vi "Inject Attribute List.vi"(6 "Attributes Ref":refnum<data-value>, 8 "error in (no error)":errorcluster, 11 "Start High Pressure Wash in":refnum<class "Start High Pressure Wash.lvclass">) -> (0 "error out":errorcluster, 3 "Start High Pressure Wash out":refnum<class "Start High Pressure Wash.lvclass">)   [LabVIEW 2019, in "Start High Pressure Wash.lvclass"]
uses:
  <vilib>/gpm_packages/@cs/Car-wash/Source/Process Steps/Start High Pressure Wash/Start High Pressure Wash.lvclass
  <vilib>/gpm_packages/@cs/lookup-table/Source/LookupTable/LookupTable.lvclass
  <vilib>/gpm_packages/@cs/lookup-table/Source/LookupTable/LookupTable.lvclass/LookupTable.ctl
  <vilib>/gpm_packages/@cs/Car-wash/Source/Process Steps/Start High Pressure Wash/Start High Pressure Wash.lvclass/Start High Pressure Wash.ctl
  203b49d5-12f0-4570-955b-2a63e2556ff9.vi
  <vilib>/gpm_packages/@cs/lookup-table/Source/LookupTable/Read Table Reference.vi
  203b49d5-12f0-4570-955b-2a63e2556ff9.vi/b3d0abb8-d302-4e7b-8dd2-78e1d69c8306.vi
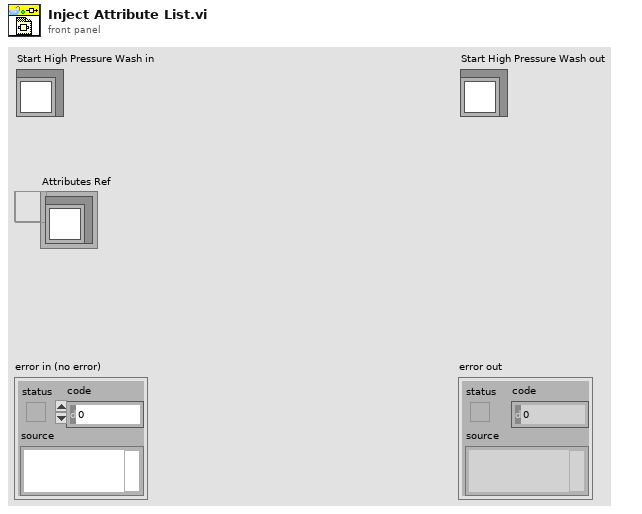
[diagram p1: front panel]
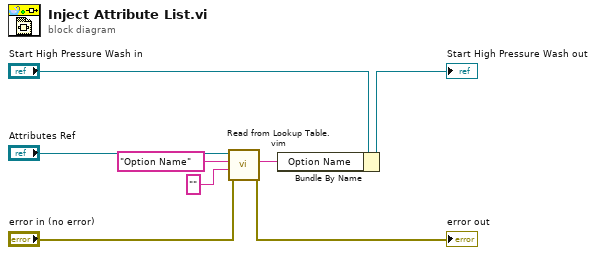
[diagram p0: block diagram]
diagram:
  n1 = call "Read from Lookup Table.vim"("error in (no error)"="error in (no error)", "Type"="", "Item Name"="Option Name", "LookupTable Reference"="Attributes Ref") -> ("error out"=→"error out":errorcluster, "Value"=w6:string)  [unwired: 4 in, 2 out]
  n2 = Bundle By Name(cluster="Start High Pressure Wash in", "Option Name"=w6) -> (→"Start High Pressure Wash out":refnum<class "Start High Pressure Wash.lvclass">)
